vi "Create_Object.vi"(8 "error in (no error)":errorcluster, 9 "Terminal Map in":map{string, T1}(c390), 10 "owner refnum":variant, 11 "MultiDiagramStructure in":refnum<class "MultiDiagramStructure.lvclass">) -> (0 "error out":errorcluster, 1 "Terminal Map Out":map{string, T1}(c390), 3 "MultiDiagramStructure out":refnum<class "MultiDiagramStructure.lvclass">)   [LabVIEW 2025, in "MultiDiagramStructure.lvclass"]
uses:
  MultiDiagramStructure.lvclass
  MultiDiagramStructure.lvclass/MultiDiagramStructure.ctl
  Node/Node.lvclass
  C:/Users/mrjak/Documents/GitHub/LVGPT/LabVIEW/VIs/Classes/Node/Node.lvclass
  C:/Users/mrjak/Documents/GitHub/LVGPT/LabVIEW/VIs/Classes/MultiDiagramStructure/MultiDiagramStructure.lvclass
  Terminal.ctl
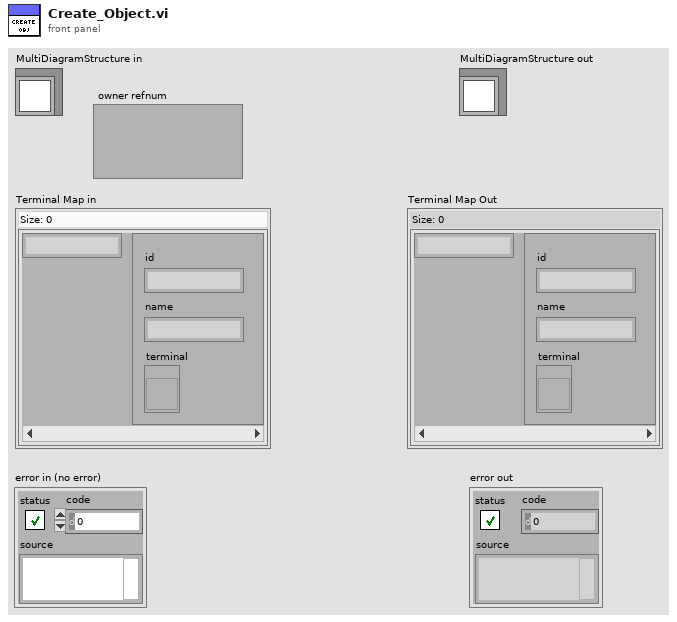
[diagram p1: front panel]
types:
  T1 = typedef "Terminal.ctl" = cluster{"id":string, "name":string, "terminal":refnum<vi>}
  T2 = typedef "LVPointTypeDef.ctl" = cluster{"Horizontal":i16, "Vertical":i16}
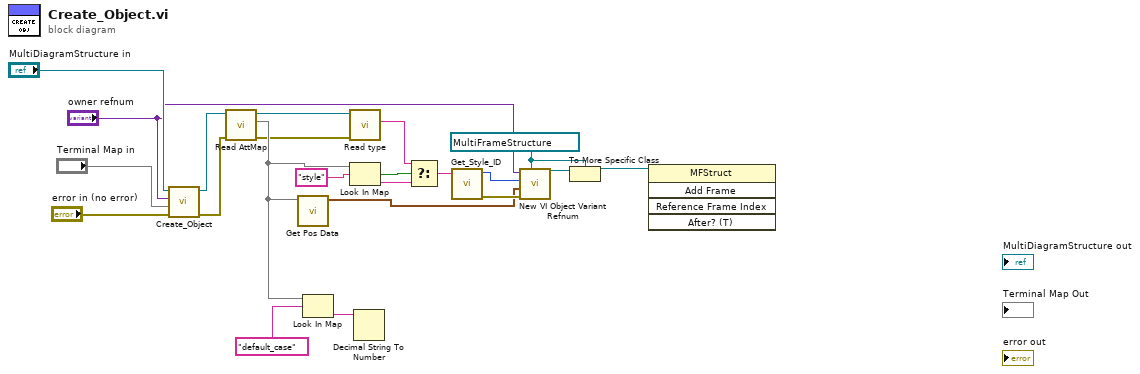
[diagram p0: block diagram]
diagram:
  w3 = refnum<vi> refnum ("vi object class")
  n1 = call-parent "Create_Object.vi"("error in (no error)"="error in (no error)", "Terminal Map in"="Terminal Map in", "owner refnum"="owner refnum", "Node in"="MultiDiagramStructure in") -> ("error out"=w20:errorcluster, "Node out"=w19:refnum<class "MultiDiagramStructure.lvclass">)  [unwired: 5 in, 1 out]
  n2 = call "Read AttMap.vi"("error in (no error)"=w20, "Node in"=w19) -> ("error out"=w7:errorcluster, "AttMap"=w9:map{string, string}, "Node out"=w8:refnum<class "MultiDiagramStructure.lvclass">)  [unwired: 7 in]
  n3 = call "Get Pos Data.vi"("AttMap"=w9) -> ("Position"=w6:T2)  [unwired: 10 in]
  n4 = Look In Map(map=w9, key="default_case") -> (value=w17:string)  [unwired: 1 in, 1 out]
  n5 = call "Read type.vi"("error in (no error)"=w7, "Node in"=w8) -> ("type"=w12:string)  [unwired: 7 in, 2 out]
  n6 = Look In Map(map=w9, key="style") -> (key not found?=w13:bool, value=w11:string)  [unwired: 1 in]
  n7 = Decimal String To Number(string=w17) -> ()  [unwired: 2 in, 2 out]
  n8 = Select(t=w12, s=w13, f=w11) -> (s? t:f=w10:string)
  n9 = call "Get_Style_ID.vi"("Style"=w10) -> ("error out"=w15:errorcluster, "style"=w16:i32)  [unwired: 8 in, 1 out]
  n10 = call "New VI Object Variant Refnum.vi"("vi object class"=w3, "error in (no error)"=w15, "location"=w6, "style"=w16, "owner refnum"="owner refnum") -> ("object refnum"=w4:refnum<vi>)  [unwired: 5 in, 1 out]
  n11 = To More Specific Class(target class=w3, reference=w4) -> (specific class reference=w2:refnum<vi>)  [unwired: 1 in, 1 out]
  n12 = invoke class="MFStruct" method="Add Frame"(reference=w2) -> (reference out=w1:refnum<vi>)  [unwired: 4 in, 4 out]
